vi "G#Debugger_ReadAttribute.vi"(0 "Subpanel dvr":refnum<data-value>, 1 "Only read attributes":bool, 5 "error in (no error)":errorcluster) -> (14 "attributes reference":refnum<vi>, 15 "attributes value":variant, 16 "valid object":bool, 17 "string":string, 18 "# of users?":i32, 19 "error out":errorcluster)   [LabVIEW 2017, in "G#Debugger.lvlib"]
uses:
  G#Debugger.lvlib
  G#Debugger_SubPanelInfo.ctl
  G#Object/G#Object.lvclass
  G#Object/utils/G#Object_ClassHierarchy.ctl
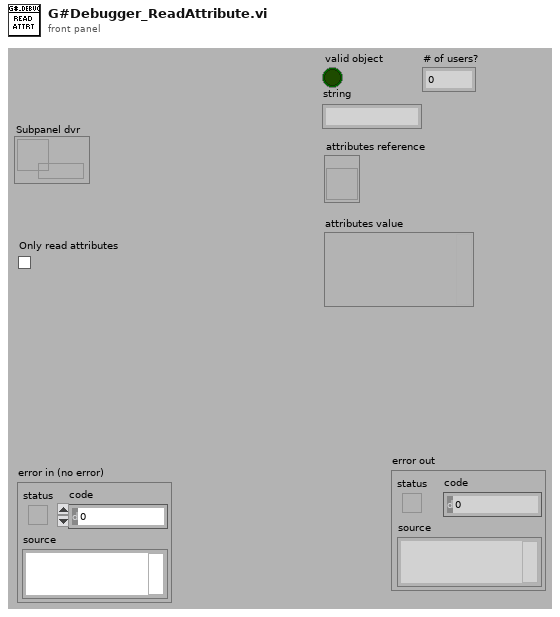
[diagram p1: front panel]
types:
  T1 = typedef "G#Debugger.lvlib/G#Debugger_SubPanelInfo.ctl" = cluster{"Ref":refnum<class "G#Object.lvclass">, "class hierarchy":T2[], "class attributes":path[], "object attributes":path[], "inheritance index":i32, "is class attributes":bool, "vi reference":refnum<vi>}
  T2 = typedef "G#Object.lvclass/G#Object_ClassHierarchy.ctl" = cluster{"ClassName":string, "FullClassName":string, "ClassPath":path, "IsLeaf":bool}
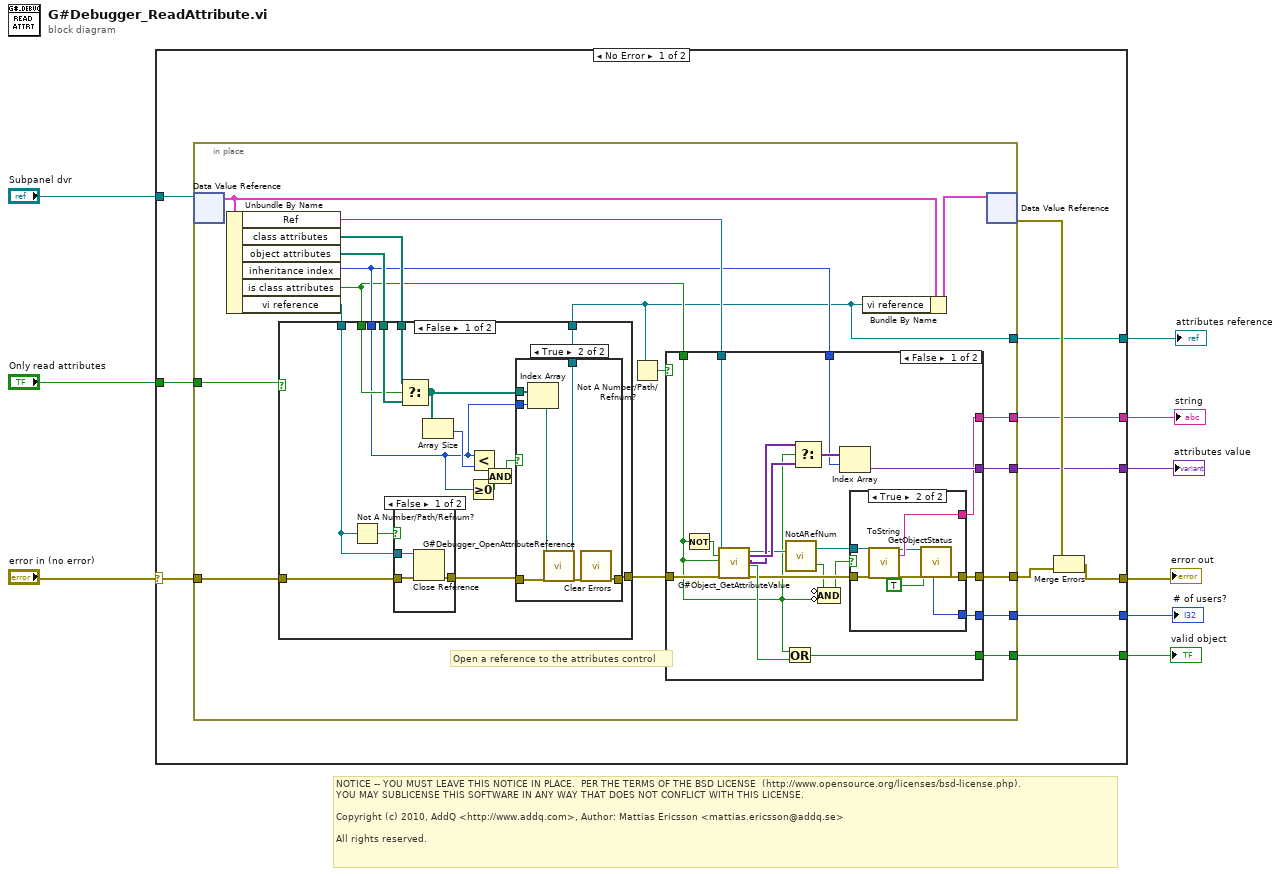
[diagram p0: block diagram]
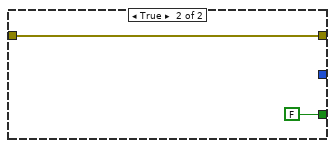
[diagram p3: hidden frame]
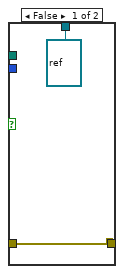
[diagram p4: hidden frame]
diagram:
  # "NOTICE -- YOU MUST LEAVE THIS NOTICE IN PLACE.  PER THE TERMS OF THE BSD LICENSE  (http://www.opensource.org/licenses/bsd-license.php).\nYOU MAY SUBLICENSE THIS SOFTWARE IN ANY WAY THAT DOES NOT CONFLICT WITH THIS LICENSE.\n\nCopyright (c) 2010, AddQ <http://www.addq.com>, Author: Mattias Ericsson <mattias.ericsson@addq.se>\n\nAll rights reserved."
  n1 = case shown="No Error" "error in (no error)" {
    selector: "error in (no error)" -> [w19 w99]
    tunnel: [w16 w99] -> w8
    tunnel: "Subpanel dvr" -> [w20 _]
    tunnel: "Only read attributes" -> [w18 _]
    tunnel: [w14 _] -> w5
    tunnel: [w13 _] -> w4
    tunnel: [w12 _] -> w3
    tunnel: [w11 _] -> w2
    tunnel: [w10 _] -> w1
    frame No Error {
      n2 = in-place {
        in-place-border: w19 -> [w36]
        in-place-border: w18 -> [w35]
        in-place-border: [w27] -> w17
        in-place-border: [w28] -> w14
        in-place-border: [w24] -> w13
        in-place-border: [w23] -> w12
        in-place-border: [w26] -> w11
        in-place-border: [w21] -> w10
        # "Open a reference to the attributes control"
        n3 = in-place-dvr #1(w20) -> (w37:T1)  [unwired: 1 out]
        n4 = Unbundle By Name(w37) -> ("Ref"=w30:refnum<class "G#Object.lvclass">, "class attributes"=w33:path[], "object attributes"=w32:path[], "inheritance index"=w29:i32, "is class attributes"=w25:bool, "vi reference"=w34:refnum<vi>)
        n5 = case shown="False" w35 {
          tunnel: w36 -> [w82 w97]
          tunnel: w34 -> [w81 w98]
          tunnel: w33 -> [w80 _]
          tunnel: w32 -> [w79 _]
          tunnel: w25 -> [w78 _]
          tunnel: w29 -> [w72 _]
          tunnel: [w76 w97] -> w31
          tunnel: [w75 w98] -> w24
          frame False {
            n6 = Not A Number/Path/Refnum?(number/path/refnum=w81) -> (NaN/Path/Refnum?=w83:bool)
            n7 = case shown="False" w83 {
              tunnel: w82 -> [w95 w96]
              tunnel: w81 -> [w94 _]
              tunnel: [w93 w96] -> w77
              frame False {
                n8 = Close Reference(reference=w94, error in (no error)=w95) -> (error out=w93:errorcluster)
              }
              frame True {
              }
            }
            n9 = Select(t=w80, s=w78, f=w79) -> (s? t:f=w74:path[])
            n10 = Array Size(array=w74) -> (size(s)=w73:i32)
            n11 = Greater Or Equal To 0?(x=w72) -> (x >= 0?=w70:bool)
            n12 = Less?(x=w72, y=w73) -> (x < y?=w71:bool)
            n13 = And(x=w71, y=w70) -> (x .and. y?=w69:bool)
            n14 = case shown="True" w69 {
              tunnel: w77 -> [w84 w92]
              tunnel: [w84 w87] -> w76
              tunnel: [refnum<vi> refnum ("vi reference") w91] -> w75
              tunnel: w74 -> [_ w90]
              tunnel: w72 -> [_ w89]
              frame False {
              }
              frame True {
                n15 = Index Array(array=w90, index=w89) -> (element=w86:path)
                n16 = call "G#Debugger_OpenAttributeReference.vi"("vi path"=w86, "error in (no error)"=w92) -> ("vi reference"=w91:refnum<vi>, "error out"=w88:errorcluster)  [unwired: 16 in]
                n17 = call <vilib>:"Clear Errors.vi"("error in (no error)"=w88) -> ("error out"=w87:errorcluster)  [unwired: 5 in, 1 out]
              }
            }
          }
          frame True {
          }
        }
        n18 = Not A Number/Path/Refnum?(number/path/refnum=w24) -> (NaN/Path/Refnum?=w22:bool)
        n19 = case shown="False" w22 {
          tunnel: w31 -> [w57 w68]
          tunnel: w30 -> [w56 _]
          tunnel: w29 -> [w54 _]
          tunnel: [w53 _] -> w28
          tunnel: [w48 w68] -> w27
          tunnel: [w47 _] -> w26
          tunnel: w25 -> [w40 _]
          tunnel: [w45 FALSE] -> w23
          tunnel: [w42 _] -> w21
          frame False {
            n20 = Not(x=w40) -> (.not. x?=w46:bool)
            n21 = call "G#Object_GetAttributeValue.vi"("reference in"=w56, "object attributes (T)"=w46, "class attributes (F)"=w40, "error in (no error)"=w57) -> ("reference out"=w44:refnum<class "G#Object.lvclass">, "attributes"=w51:variant[], "class attributes"=w50:variant[], "valid object"=w52:bool, "error out"=w49:errorcluster)  [unwired: 11 in]
            n22 = Or(x=w40, y=w52) -> (x .or. y?=w45:bool)
            n23 = call-dynamic "NotARefNum.vi"("reference in"=w44) -> ("not a refnum?"=w41:bool, "reference out"=w43:refnum<class "G#Object.lvclass">)  [unwired: 1 in]
            n24 = Select(t=w50, s=w40, f=w51) -> (s? t:f=w55:variant[])
            n25 = Compound Arithmetic op=AND(invert w41, invert w40) -> (w39:bool)
            n26 = Index Array(array=w55, index=w54) -> (element=w53:variant)
            n27 = case shown="True" w39 {
              tunnel: w49 -> [w58 w66]
              tunnel: [w58 w62] -> w48
              tunnel: [_ w65] -> w47
              tunnel: w43 -> [_ w64]
              tunnel: [_ w59] -> w42
              frame False {
              }
              frame True {
                n28 = call-dynamic "ToString.vi"("reference in"=w64, "error in (no error)"=w66) -> ("reference out"=w61:refnum<class "G#Object.lvclass">, "string"=w65:string, "error out"=w63:errorcluster)  [unwired: 15 in]
                n29 = call-dynamic "GetObjectStatus.vi"("reference in"=w61, "simple info (F)"=TRUE, "error in (no error)"=w63) -> ("# of users?"=w59:i32, "error out"=w62:errorcluster)  [unwired: 5 in, 10 out]
              }
            }
          }
          frame True {
          }
        }
        n30 = Bundle By Name(cluster=w37, "vi reference"=w24) -> (w38:T1)
        n31 = in-place-dvr #1(w38) -> (w15:errorcluster)  [unwired: 1 out]
      }
      n32 = Merge Errors(w15, w17) -> (w16:errorcluster)
    }
    frame Error {
    }
  }
  "error out" <- w8
  "attributes value" <- w5
  "attributes reference" <- w4
  "valid object" <- w3
  "string" <- w2
  "# of users?" <- w1
